vi "New Image (Greyscale Array).vi"(8 "error in (no error)":errorcluster, 11 "U8 Greyscale Data":u8[][](array[numeric])) -> (0 "error out":errorcluster, 3 "Greyscale Image":T1)   [LabVIEW 2020, in "image.lvlib"]
doc: "Create a New Image. The New Image data can be prep-populated with the given array of U8 image data.\n\nTo create a New Image which has a preallocated size with a uniform value, use the \"New Image (Greyscale Preallocated).vi\""
uses:
  image.lvlib
  Greyscale Image.ctl
  common/common.lvlib
  common/bin/gartoolkit_32-1.dll
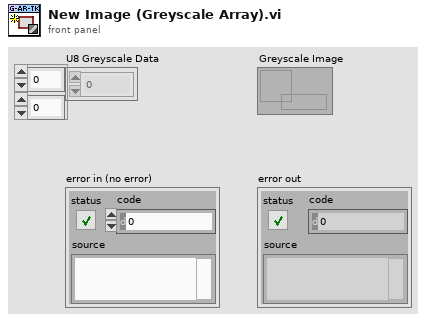
[diagram p1: front panel]
types:
  T1 = typedef "image.lvlib/Greyscale Image.ctl" = refnum<data-value>
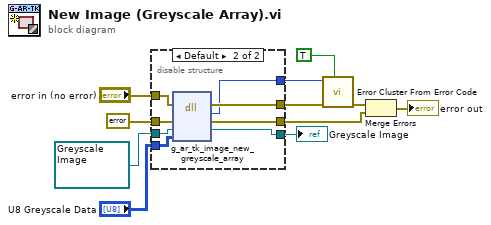
[diagram p0: block diagram]
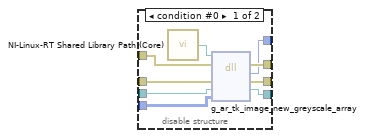
[diagram p2: hidden frame]
diagram:
  n1 = disable-structure shown="Default" {
    disable-tunnel: errorcluster {"status"=FALSE, "code"=0, "source"=""} ("error constant") -> [w20 w28]
    disable-tunnel: T1 refnum ("Ref Type") -> [w19 w27]
    disable-tunnel: "U8 Greyscale Data" -> [w18 w26]
    disable-tunnel: [w17 w25] -> w6
    disable-tunnel: [w16 w24] -> w5
    disable-tunnel: [w15 w23] -> w4
    disable-tunnel: [w14 w22] -> w3
    disable-tunnel: "error in (no error)" -> [w12 w21]
    frame condition #0 {
      n2 = call "NI-Linux-RT Shared Library Path (Core).vi"() -> ("Path"=w13:path)
      n3 = dll-call lib="?" fn="g_ar_tk_image_new_greyscale_array" ("g_ar_toolkit.*.*:g_ar_tk_image_create")(path in=w13, error in=w12, "error_cluster"=w20, "EDVR"=w19, "array_handle"=w18) -> (error out=w17:errorcluster, w16:i32, "error_cluster"=w15:errorcluster, "EDVR"=w14:T1)  [unwired: 2 in, 1 out]
    }
    frame condition #1 (active) {
      n4 = dll-call lib="C:/serenial/lib/g-augmented-reality-toolkit/LabVIEW/common/bin/gartoolkit_*-1.*" fn="g_ar_tk_image_new_greyscale_array" ("g_ar_toolkit.*.*:g_ar_tk_image_create")(error in=w21, "error_cluster"=w28, "EDVR"=w27, "array_handle"=w26) -> (error out=w25:errorcluster, w24:i32, "error_cluster"=w23:errorcluster, "EDVR"=w22:T1)  [unwired: 3 in, 1 out]
    }
  }
  "Greyscale Image" <- w3
  n5 = call <vilib>:"Error Cluster From Error Code.vi"("show call chain? (False)"=TRUE, "error in (no error)"=w6, "error code (0)"=w5) -> ("error out"=w10:errorcluster)  [unwired: 6 in]
  n6 = Merge Errors(w10, w4) -> (→"error out":errorcluster)
